vi "Autoshutter.vi"(0 "Autoshutter Steps":enum32{"Relative", "Absolute"}(ring), 4 "%":dbl=10.0, 5 "Autoshutter Limits":cluster{"Upper Limit":i32, "Lopwer Limit":i32}, 6 "error in":errorcluster, 7 "Session in":T2, 8 "Global Report":T1, 9 "Autoshutter Value":dbl, 10 "ms":dbl=10.0) -> (2 "error out":errorcluster, 3 "Session Out":T2)   [LabVIEW 2009]
uses:
  <vilib>/userDefined/High Color/IMAQdx.ctl
  Program Files/National Instruments/LabVIEW 2009/resource/objmgr/imaqdx.rc
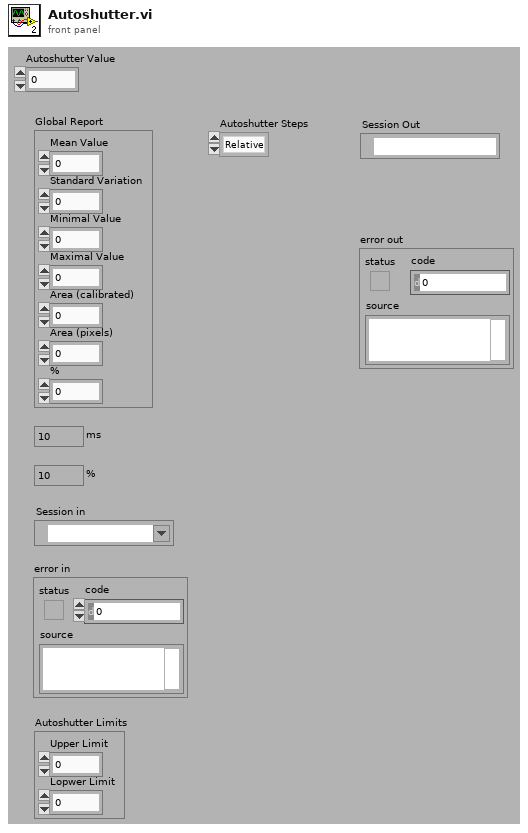
[diagram p1: front panel]
types:
  T1 = cluster{"Mean Value":sgl, "Standard Variation":sgl, "Minimal Value":sgl, "Maximal Value":sgl, "Area (calibrated)":sgl, "Area (pixels)":i32, "%":sgl}
  T2 = typedef "IMAQdx.ctl" = refnum<k21>
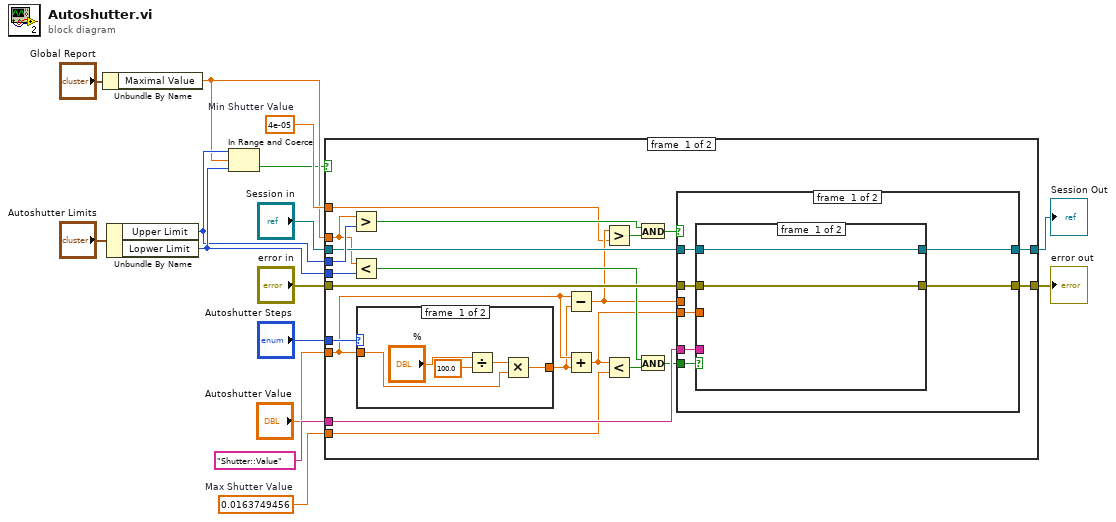
[diagram p0: block diagram]
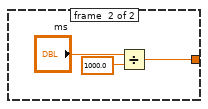
[diagram p2: hidden frame]
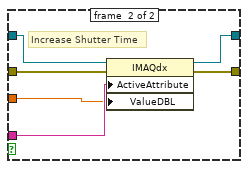
[diagram p3: hidden frame]
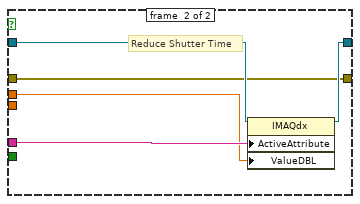
[diagram p4: hidden frame]
diagram:
  w11 = 4e-05  # Min Shutter Value
  w14 = 0.0163749456  # Max Shutter Value
  n1 = Unbundle By Name("Global Report") -> ("Maximal Value"=w7:sgl)
  n2 = Unbundle By Name("Autoshutter Limits") -> ("Upper Limit"=w8:i32, "Lopwer Limit"=w10:i32)
  n3 = In Range and Coerce(upper limit=w8, x=w7, lower limit=w10) -> (In Range?=w6:bool)  [unwired: 1 out]
  n4 = case shown="False" w6 {
    tunnel: w7 -> [w31 _]
    tunnel: w8 -> [w36 _]
    tunnel: "Session in" -> [w35 w66]
    tunnel: "error in" -> [w34 w65]
    tunnel: [w33 w66] -> w12
    tunnel: "Autoshutter Value" -> [w20 _]
    tunnel: "Shutter::Value" ("ActiveAttribute") -> [w32 _]
    tunnel: w10 -> [w30 _]
    tunnel: [w29 w65] -> w13
    tunnel: w11 -> [w22 _]
    tunnel: w14 -> [w18 _]
    tunnel: "Autoshutter Steps" -> [w25 _]
    frame #0 {
      n5 = Greater?(x=w31, y=w36) -> (0:w24:bool)
      n6 = Less?(x=w31, y=w30) -> (x < y?=w26:bool)
      n7 = case shown="\"Relative\", Default" w25 {
        tunnel: w20 -> [w38 _]
        tunnel: [w37 w42] -> w19
        frame #0 {
          n8 = Divide(x="%", y=100.0) -> (x/y=w39:dbl)
          n9 = Multiply(x=w39, y=w38) -> (x*y=w37:dbl)
        }
        frame #1 {
          n10 = Divide(x="ms", y=1000.0) -> (x/y=w42:dbl)
        }
      }
      n11 = Subtract(x=w20, y=w19) -> (x-y=w23:dbl)
      n12 = Add(x=w20, y=w19) -> (x+y=w16:dbl)
      n13 = Greater?(x=w23, y=w22) -> (0:w21:bool)
      n14 = Less?(x=w16, y=w18) -> (x < y?=w17:bool)
      n15 = And(x=w24, y=w21) -> (x .and. y?=w28:bool)
      n16 = And(x=w26, y=w17) -> (x .and. y?=w27:bool)
      n17 = case shown="True" w28 {
        tunnel: w35 -> [w51 w64]
        tunnel: w34 -> [w47 w61]
        tunnel: [w50 w63] -> w33
        tunnel: w32 -> [w49 w62]
        tunnel: w27 -> [w48 _]
        tunnel: [w46 w61] -> w29
        tunnel: w23 -> [_ w60]
        tunnel: w16 -> [w45 _]
        frame #0 {
          n18 = case shown="True" w48 {
            tunnel: w51 -> [w53 w59]
            tunnel: [w53 w58] -> w50
            tunnel: w49 -> [_ w57]
            tunnel: w47 -> [w52 w56]
            tunnel: [w52 w55] -> w46
            tunnel: w45 -> [_ w54]
            frame #0 {
            }
            frame #1 {
              # "Increase Shutter Time"
              n19 = property class="IMAQdx"(reference=w59, error in=w56, "ActiveAttribute"=w57, "ValueDBL"=w54) -> (reference out=w58:T2, error out=w55:errorcluster)
            }
          }
        }
        frame #1 {
          # "Reduce Shutter Time"
          n20 = property class="IMAQdx"(reference=w64, "ActiveAttribute"=w62, "ValueDBL"=w60) -> (reference out=w63:T2)  [unwired: 1 in, 1 out]
        }
      }
    }
    frame #1 {
    }
  }
  "error out" <- w13
  "Session Out" <- w12
